vi "Launch.vi"() -> (3 "Data Generator API.lvclass":refnum<class "Data Generator API.lvclass">)   [LabVIEW 2024, in "Data Generator Actor.lvclass"]
uses:
  Data Generator Actor.lvclass
  Data Generator API/Data Generator API.lvclass
  C:/Users/320141162/Desktop/DUTLug3/API/API.lvclass
  Core.vi
panel:
  out "error out":errorcluster
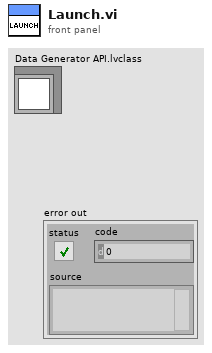
[diagram p1: front panel]
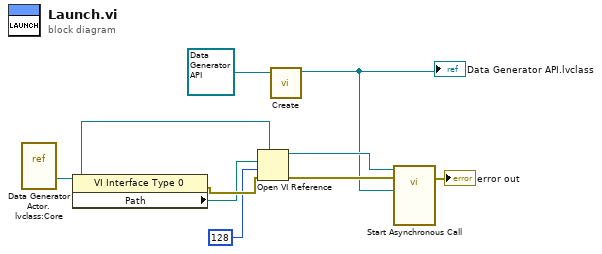
[diagram p0: block diagram]
diagram:
  n1 = vi-ref "Data Generator Actor.lvclass:Core.vi"() -> (w4:refnum<vi>)
  n2 = property class="VI Interface Type 0"(reference=w4) -> (error out=w8:errorcluster, "Path"=w7:path)  [unwired: 1 in, 1 out]
  n3 = Open VI Reference(type specifier VI Refnum (for type only)=w4, vi path=w7, options=128, error in (no error)=w8) -> (vi reference=w5:refnum<vi>, error out=w6:errorcluster)  [unwired: 2 in]
  n4 = call-dynamic "Create.vi"("API out 2"=refnum<class "Data Generator API.lvclass"> refnum ("Data Generator API.lvclass")) -> ("API out"=w3:refnum<class "Data Generator API.lvclass">)  [unwired: 10 in]
  "Data Generator API.lvclass" <- w3
  n5 = call-by-ref "Start Asynchronous Call"(reference=w5, error in=w6, "API.lvclass"=w3) -> (error out=→"error out":errorcluster)  [unwired: 9 in, 3 out]
